vi "PV Miscellaneous.vi"(8 "error in (no error)":errorcluster, 9 "PV Miscellaneous - Cluster":T1={"Parameter"=enum." Preselection brake", "Parameter\nread only<->describe"=FALSE, "off<->on   "=TRUE, "Unit adress"=1, "Contens of service\nline; # of the 2nd\n parameter"=795} {"Contens of service\nline; # of the 2nd\n parameter" min=0 max=999 step=1; "Unit adress" min=1 max=255 step=1}, 10 "Adress of unit":u16=1 max=999 step=1, 11 "VISA session":refnum<visa-resource-name>) -> (0 "error out":errorcluster, 2 "response (data)":string, 3 "dup VISA session":refnum<visa-resource-name>)   [LabVIEW 2024, in "Pfeiffer Vacuum.lvlib"]
doc: "There are 12 parameters available, only one of which can be enabled at a time. \n\nPreselection brake (default) (013)\nRemote operations mode (028)\nActual error code (read only) (303)\nSoftware version electronic drive unit (read only) (312)\nSoftware version display and control unit (read only) (351)\nParameter set (794)\nContens of service line (TCM 1601 only) (795)\nUnit adress (797)\nUnit type electronic drive unit (349)\nError acknowledgement (write only) (009)\nKeyboard interlock (008)\nSeal gas enable (050)\n\nNote: Any settings for an parameter that is not selected will be ignored. If a value is out of range, it will be changed to either the upper or the lower limit of the range."
uses:
  <instrlib>/Pfeiffer Vacuum/Pfeiffer Vacuum.lvlib
  <instrlib>/Pfeiffer Vacuum/Public/Turbopumps/PV Miscellaneous - Cluster.ctl
panel:
  # "Preselection brake             :  \n Remote operations mode  : \n Configuration output K4    : \n Parameter set                      :\n Seal gas enable                   :\n Keyboard interlock            :"
  # "<--------------\n  off\n  stand. operations \n  heat/TMS\n  basic  \n  off\n  off"
  # "----------->          \non \nremote priority \nPWM-signal \n extended \non \non"
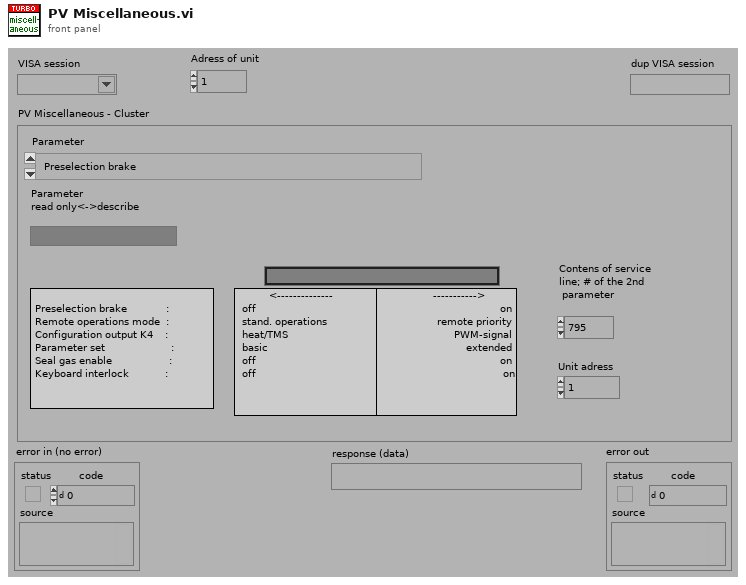
[diagram p1: front panel]
types:
  T1 = typedef "Pfeiffer Vacuum.lvlib/PV Miscellaneous - Cluster.ctl" = cluster{"Parameter":enum16{" Preselection brake", " Remote operations mode", " Actual error code (read only)", " Software version electronic drive unit  (read only)", " Software version display and control unit  (read only)", " Parameter set", " Contens of service line (TCM 1601 only)", " Unit adress", " Unit type electronic drive unit", " Error acknowledgement (write only)", " Keyboard interlock (008)", " Seal gas enable (050)"}, "Parameter\nread only<->describe":bool, "off<->on   ":bool, "Unit adress":i16, "Contens of service\nline; # of the 2nd\n parameter":i16}
  T2 = enum16{" Preselection brake", " Remote operations mode", " Actual error code (read only)", " Software version electronic drive unit  (read only)", " Software version display and control unit  (read only)", " Parameter set", " Contens of service line (TCM 1601 only)", " Unit adress", " Unit type electronic drive unit", " Error acknowledgement (write only)", " Keyboard interlock (008)", " Seal gas enable (050)"}
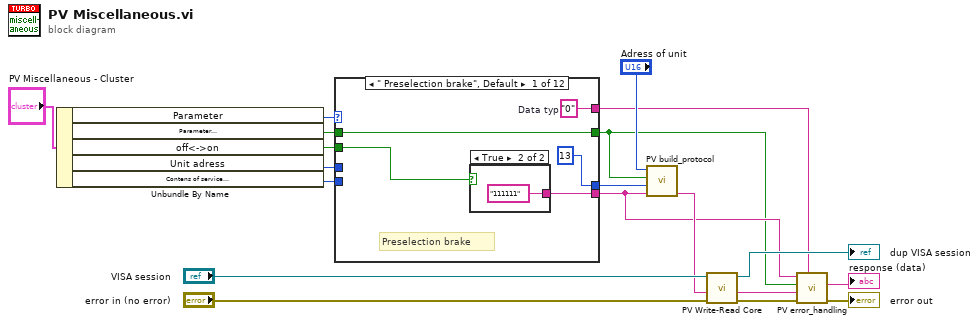
[diagram p0: block diagram]
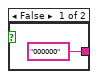
[diagram p2: hidden frame]
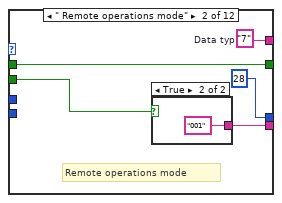
[diagram p3: hidden frame]
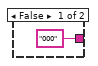
[diagram p4: hidden frame]
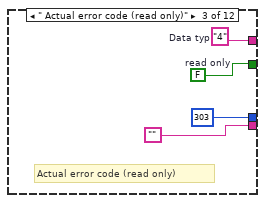
[diagram p5: hidden frame]
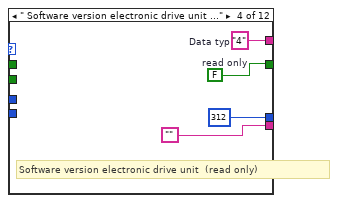
[diagram p6: hidden frame]
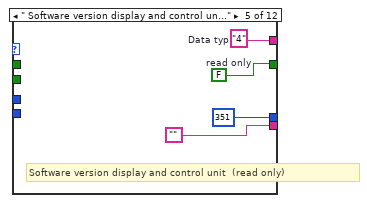
[diagram p7: hidden frame]
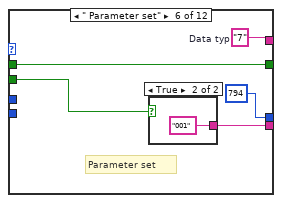
[diagram p8: hidden frame]
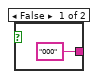
[diagram p9: hidden frame]
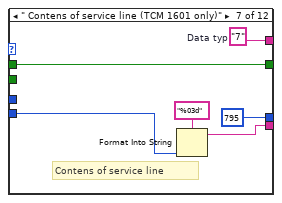
[diagram p10: hidden frame]
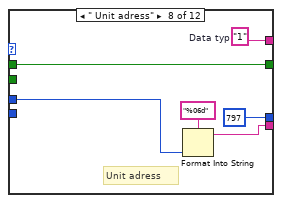
[diagram p11: hidden frame]
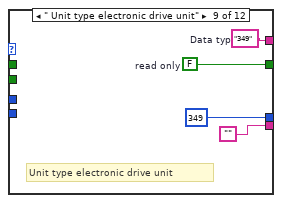
[diagram p12: hidden frame]
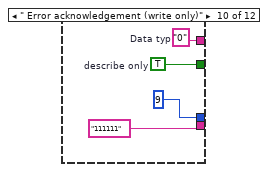
[diagram p13: hidden frame]
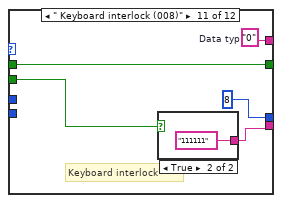
[diagram p14: hidden frame]
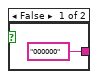
[diagram p15: hidden frame]
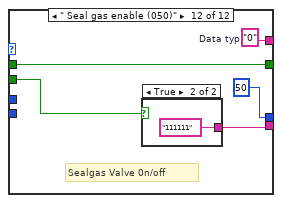
[diagram p16: hidden frame]
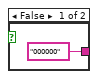
[diagram p17: hidden frame]
diagram:
  n1 = Unbundle By Name("PV Miscellaneous - Cluster") -> ("Parameter"=w17:T2, "Parameter\nread only<->describe"=w16:bool, "off<->on"=w14:bool, "Unit adress"=w13:i16, "Contens of service\nline; # of the 2nd\n parameter"=w12:i16)
  n2 = case shown="\" Preselection brake\", Default" w17 {
    tunnel: [u16 13 ("Parameter-number") u16 28 ("Parameter-number") u16 303 ("Parameter-number") u16 312 ("Parameter-number") u16 351 ("Parameter-number") u16 794 ("Parameter-number") u16 795 ("Parameter-number") u16 797 ("Parameter-number") u16 349 ("Parameter-number") u16 9 ("Parameter-number") u16 8 ("Parameter-number") u16 50 ("Parameter-number")] -> w18
    tunnel: [w23 w30 "" "" "" w49 w57 w63 "" "111111" ("Data") w73 w81] -> w4
    tunnel: [w22 w29 w36 w40 w44 w48 w55 w61 w68 w72 w75 w83] -> w3
    tunnel: w16 -> [w22 w29 _ _ _ w48 w55 w61 _ _ w75 w83]
    tunnel: w14 -> [w21 w28 _ _ _ w47 _ _ _ _ w74 w82]
    tunnel: w13 -> [_ _ _ _ _ _ _ w60 _ _ _ _]
    tunnel: w12 -> [_ _ _ _ _ _ w54 _ _ _ _ _]
    tunnel: [w20 w27 w34 w38 w42 w46 w53 w59 w65 w69 w76 w84] -> w5
    frame " Preselection brake", Default {
      w20 = "0"  # Data typ
      # "Preselection brake"
      n3 = case shown="True" w21 {
        tunnel: ["000000" ("Data") "111111" ("Data")] -> w23
        frame False {
        }
        frame True {
        }
      }
    }
    frame " Remote operations mode" {
      w27 = "7"  # Data typ
      # "Remote operations mode"
      n4 = case shown="True" w28 {
        tunnel: ["000" ("Data") "001" ("Data")] -> w30
        frame False {
        }
        frame True {
        }
      }
    }
    frame " Actual error code (read only)" {
      w34 = "4"  # Data typ
      w36 = FALSE  # read only
      # "Actual error code (read only)"
    }
    frame " Software version electronic drive unit  (read only)" {
      w38 = "4"  # Data typ
      w40 = FALSE  # read only
      # "Software version electronic drive unit  (read only)"
    }
    frame " Software version display and control unit  (read only)" {
      w42 = "4"  # Data typ
      w44 = FALSE  # read only
      # "Software version display and control unit  (read only)"
    }
    frame " Parameter set" {
      w46 = "7"  # Data typ
      # "Parameter set"
      n5 = case shown="True" w47 {
        tunnel: ["000" ("Data") "001" ("Data")] -> w49
        frame False {
        }
        frame True {
        }
      }
    }
    frame " Contens of service line (TCM 1601 only)" {
      w53 = "7"  # Data typ
      # "Contens of service line"
      n6 = Format Into String(format string="%03d" ("Format-String"), w54) -> (resulting string=w57:string)  [unwired: 2 in, 1 out]
    }
    frame " Unit adress" {
      w59 = "1"  # Data typ
      # "Unit adress"
      n7 = Format Into String(format string="%06d" ("Format-String"), w60) -> (resulting string=w63:string)  [unwired: 2 in, 1 out]
    }
    frame " Unit type electronic drive unit" {
      w65 = "349"  # Data typ
      w68 = FALSE  # read only
      # "Unit type electronic drive unit"
    }
    frame " Error acknowledgement (write only)" {
      w69 = "0"  # Data typ
      w72 = TRUE  # describe only
    }
    frame " Keyboard interlock (008)" {
      w76 = "0"  # Data typ
      # "Keyboard interlock"
      n8 = case shown="True" w74 {
        tunnel: ["000000" ("Data") "111111" ("Data")] -> w73
        frame False {
        }
        frame True {
        }
      }
    }
    frame " Seal gas enable (050)" {
      w84 = "0"  # Data typ
      # "Sealgas Valve 0n/off"
      n9 = case shown="True" w82 {
        tunnel: ["000000" ("Data") "111111" ("Data")] -> w81
        frame False {
        }
        frame True {
        }
      }
    }
  }
  n10 = call <instrlib>:"PV build_protocol.vi"("Data"=w4, "Parameter-number"=w18, "parameter\nread<->describe"=w3, "Adress"="Adress of unit") -> ("output"=w9:string)  [unwired: 3 in]
  n11 = call <instrlib>:"PV Write-Read Core.vi"("error in"="error in (no error)", "Write data in"=w9, "VISA session"="VISA session") -> ("error out"=w6:errorcluster, "response (data) out"=w7:string, "dup VISA session"=→"dup VISA session":refnum<visa-resource-name>)  [unwired: 2 in]
  n12 = call <instrlib>:"PV error_handling.vi"("Data Typ in"=w5, "error in"=w6, "response (data) in"=w7, "Parameter\nread only<->describe"=w3, "data in"=w4) -> ("error out"=→"error out":errorcluster, "Data out"=→"response (data)":string)  [unwired: 4 in, 1 out]
